vi "plot_example_XY.vi"() -> ()   [LabVIEW 2010, in "OSA.lvclass"]
doc: "Example for plotting XY data, with data reduction, (10E6 XY pairs reduced to graph pixel X-size)."
uses:
  OSA.lvclass
  <vilib>/measure/NI_MABase.lvlib
  typeDef/acq_dataType.ctl
  _misc/Thorlabs_FTS_misc.llb/graph_spectrum.ctl
  OSA20X_misc.lvlib
panel:
  in  "exit butt":bool
  in  "ZOOM OUT BUTTON":bool
  in  "PANE RIGHT":bool
  in  "PANE LEFT":bool
  in  "ZOOM RESTORE":bool
  in  "ZOOM IN BUTTON":bool
  out "Intensity Graph spectrum":T1
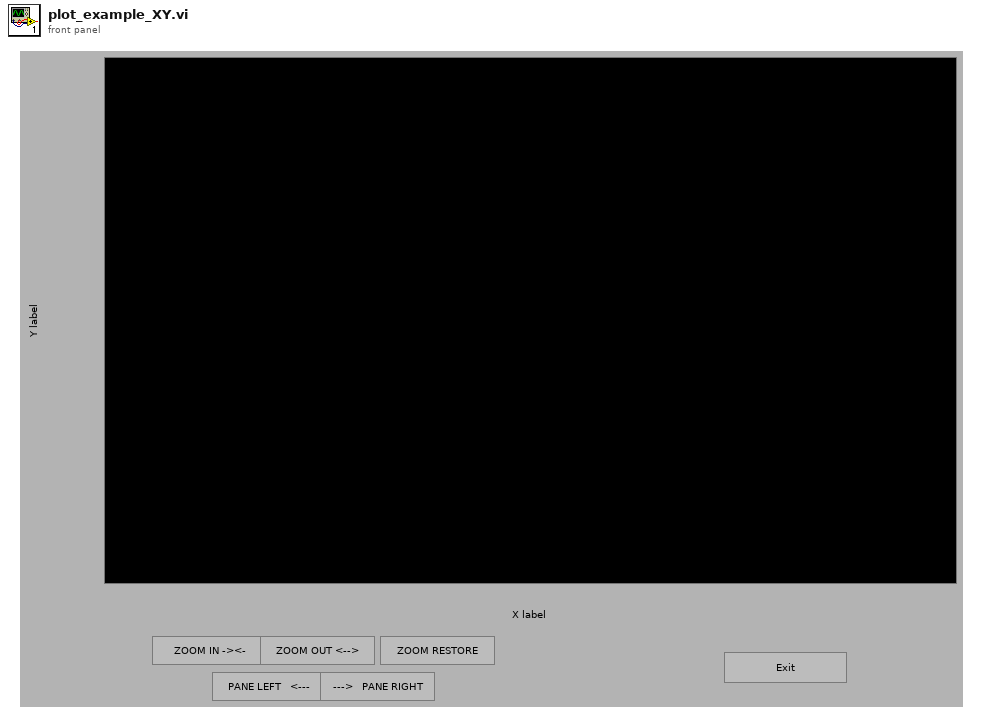
[diagram p1: front panel]
types:
  T1 = typedef "OSA20X_misc.lvlib/graph_spectrum.ctl" = i32[][]
  T2 = typedef "OSA.lvclass/acq_dataType.ctl" = enum16{"none", "interferogram", "spectrum"}
  T3 = enum16{"user", "cursor", "mouse", "pane", "reset"}
  T4 = enum16{"user", "cursor", "mouse", "pane", "reset", "pane right", "zoom out"}
  T5 = enum16{"user", "cursor", "mouse", "pane", "reset", "pane right"}
  T6 = typedef "LVPoint32TypeDef.ctl" = cluster{"Horizontal":i32, "Vertical":i32}
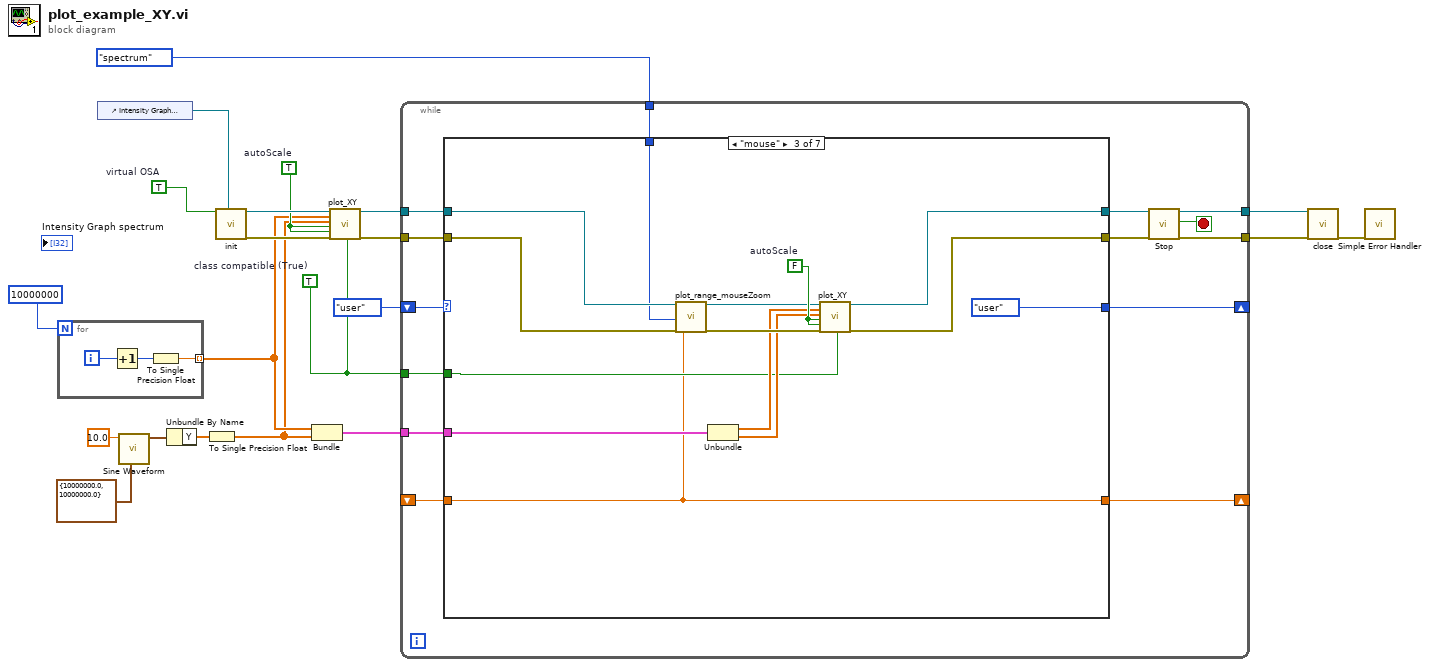
[diagram p0: block diagram]
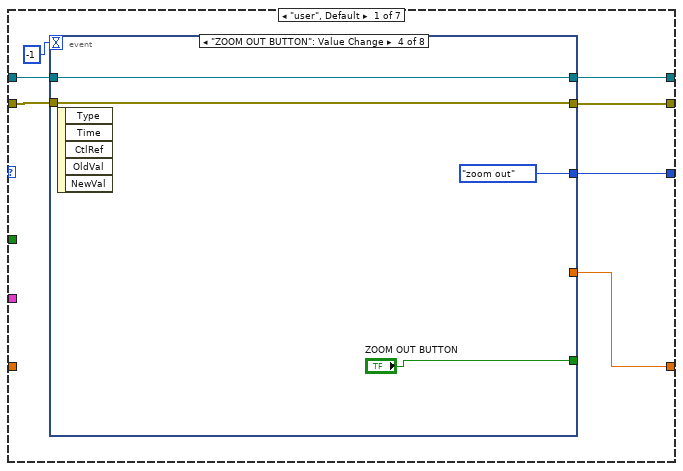
[diagram p2: hidden frame]
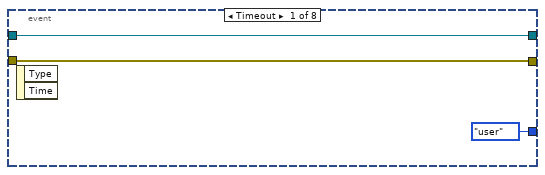
[diagram p3: hidden frame]
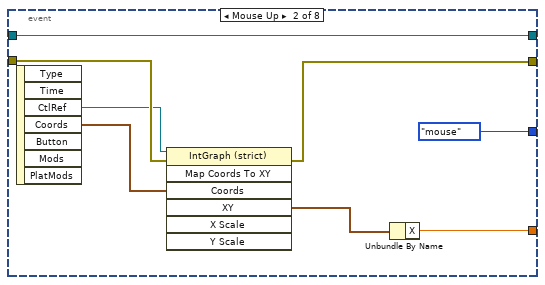
[diagram p4: hidden frame]
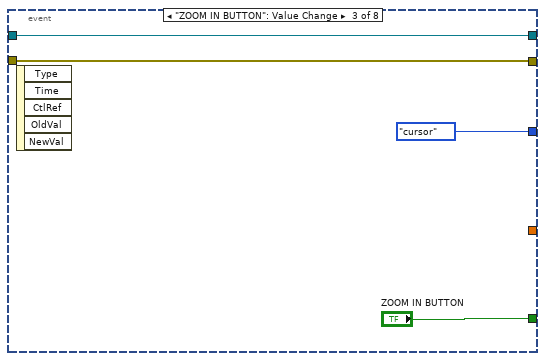
[diagram p5: hidden frame]
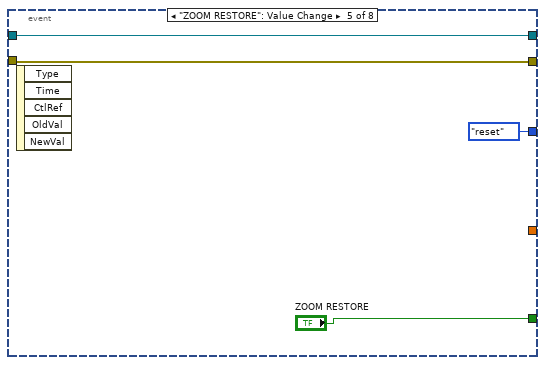
[diagram p6: hidden frame]
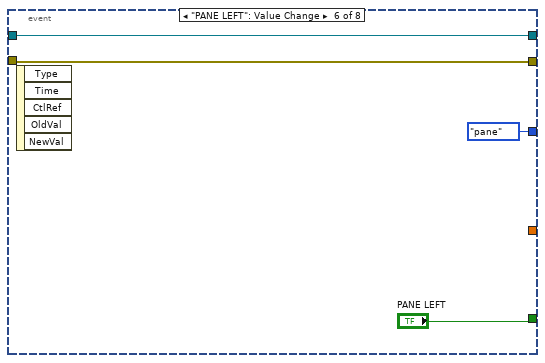
[diagram p7: hidden frame]
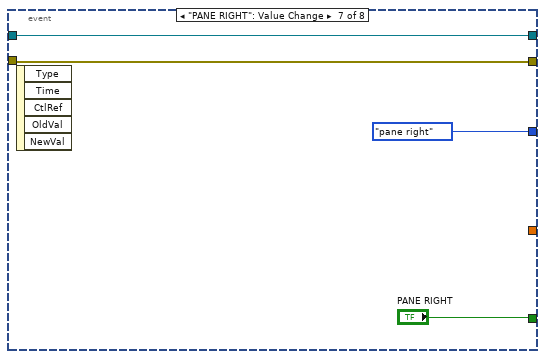
[diagram p8: hidden frame]
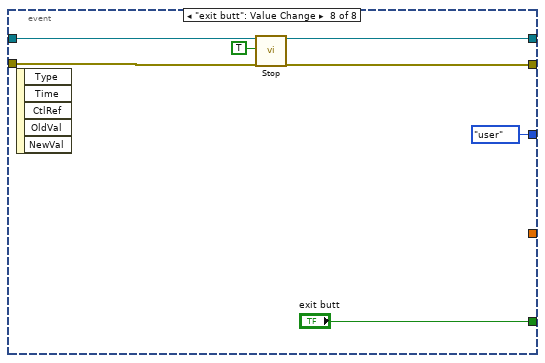
[diagram p9: hidden frame]
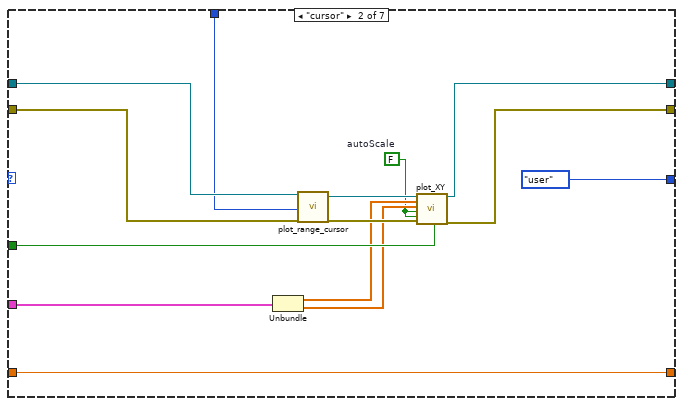
[diagram p10: hidden frame]
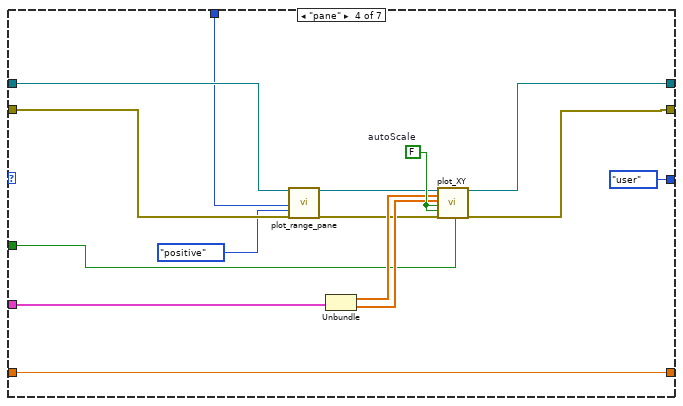
[diagram p11: hidden frame]
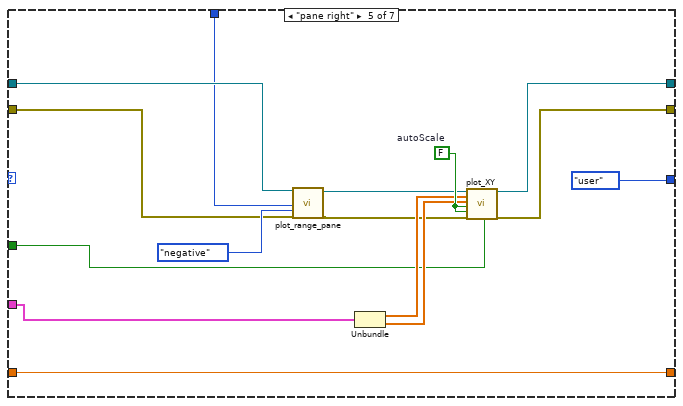
[diagram p12: hidden frame]
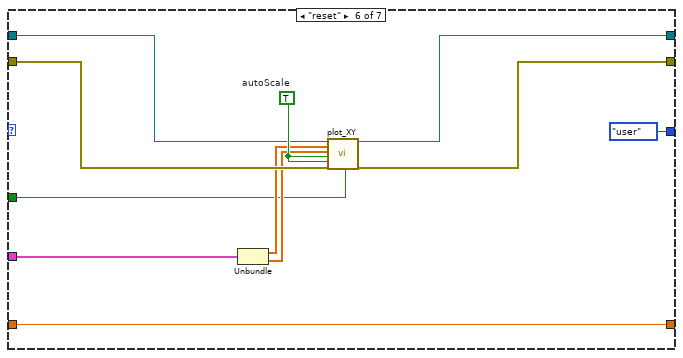
[diagram p13: hidden frame]
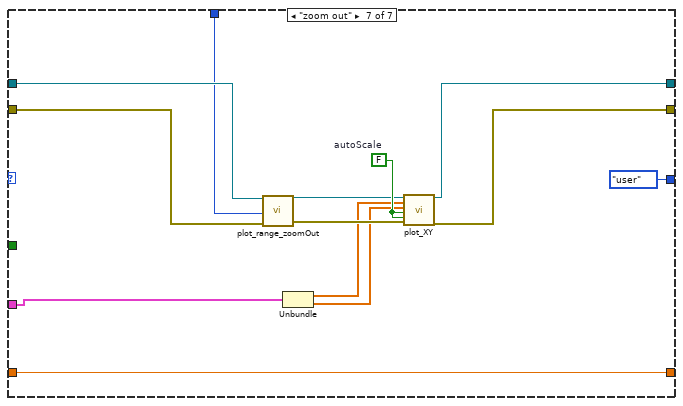
[diagram p14: hidden frame]
diagram:
  w6 = TRUE  # class compatible (True)
  w7 = TRUE  # autoScale
  w19 = TRUE  # virtual OSA
  n1 = for {
    N: 10000000 -> [_]
    tunnel: [w23] -> w5 mode=indexing
    i -> [w24]
    n2 = Increment(x=w24) -> (x+1=w22:i32)
    n3 = To Single Precision Float(number=w22) -> (single precision float=w23:sgl)
  }
  n4 = control-ref of="Intensity Graph spectrum"() -> (w18:refnum<vi>)
  n5 = call <vilib>:"Sine Waveform.vi"("sampling info"=cluster{"Fs":dbl, "#s":dbl} {"Fs"=10000000.0, "#s"=10000000.0}, "frequency"=10.0) -> ("signal out"=w16:waveform(dbl))  [unwired: 8 in, 1 out]
  n6 = Unbundle By Name(w16) -> ("Y"=w12:dbl[])
  n7 = To Single Precision Float(number=w12) -> (single precision float=w4:sgl[])
  n8 = call "init.vi"("virtual OSA"=w19, "Graph Spectrum"=w18) -> ("duplicate reference"=w21:refnum<class "OSA.lvclass">, "error out"=w20:errorcluster)  [unwired: 13 in, 3 out]
  n9 = Bundle(w5, w4) -> (w3:cluster{sgl[], sgl[]})  [unwired: 1 in]
  n10 = call "plot_XY.vi"("reference"=w21, "X-data"=w5, "Y-data"=w4, "autoScale X (True)"=w7, "autoScale Y (True)"=w7, "error in (no error)"=w20, "class compatible (True)"=w6) -> ("duplicate reference"=w11:refnum<class "OSA.lvclass">, "error out"=w10:errorcluster)  [unwired: 11 in]
  n11 = while {
    shift-right: [w37] -> _
    shift-left: T3."user" -> [w38]
    tunnel: w11 -> [w36]
    tunnel: w10 -> [w35]
    tunnel: [w26] -> w9
    tunnel: [w27] -> w8
    tunnel: w6 -> [w34]
    tunnel: w3 -> [w33]
    tunnel: acq_dataType."spectrum" ("dataType") -> [w32]
    shift-right: [w31] -> _
    shift-left: _ -> [w30]
    stop <- w25 stop-if-true
    n12 = case shown="\"mouse\"" w38 {
      tunnel: [w44 T3."user" T3."user" T3."user" T3."user" T5."user" T4."user"] -> w37
      tunnel: w36 -> [w40 w97 w109 w125 w140 w151 w165]
      tunnel: w35 -> [w43 w96 w110 w126 w139 w148 w164]
      tunnel: [w42 w94 w102 w113 w131 w149 w159] -> w28
      tunnel: [w39 w92 w101 w114 w132 w150 w160] -> w29
      tunnel: w34 -> [_ w90 w100 w112 w127 w142 _]
      tunnel: w33 -> [_ w91 w105 w117 w128 w147 w156]
      tunnel: w32 -> [_ w85 w106 w123 w138 _ w162]
      tunnel: [w41 w84 w98 w121 w137 w143 w153] -> w31
      tunnel: w30 -> [_ w84 w98 w121 w137 w143 w153]
      frame "user", Default {
        n13 = event shown="[3] \"ZOOM OUT BUTTON\": Value Change" {
          selector: _ -> [_ _ _ _ _ _ _ _]
          dyn-events: _ -> [_ _ _ _ _ _ _ _]
          timeout: -1 -> [_ _ _ _ _ _ _ _]
          tunnel: [T3."user" T3."mouse" T3."cursor" T4."zoom out" T5."reset" T3."pane" T5."pane right" T3."user"] -> w44
          tunnel: w43 -> [w47 w54 w59 w63 w65 w70 w74 w82]
          tunnel: [w47 w53 w59 w63 w65 w70 w74 w81] -> w42
          tunnel: [_ w51 _ _ _ _ _ _] -> w41
          tunnel: w40 -> [w46 w49 w58 w62 w66 w71 w75 w83]
          tunnel: [w46 w49 w58 w62 w66 w71 w75 w80] -> w39
          tunnel: [_ _ "ZOOM IN BUTTON" "ZOOM OUT BUTTON" "ZOOM RESTORE" "PANE LEFT" "PANE RIGHT" "exit butt"] -> _
          event Timeout {
            n14 = event-data() -> ()  [unwired: 1 in, 2 out]
          }
          event Mouse Up {
            n15 = event-data() -> ("CtlRef"=w50:refnum<vi>, "Coords"=w55:T6)  [unwired: 1 in, 5 out]
            n16 = invoke class="IntGraph (strict)" method="Map Coords To XY"(reference=w50, error in=w54, "Coords"=w55) -> (error out=w53:errorcluster, "XY"=w52:cluster{"X":dbl, "Y":dbl})  [unwired: 4 in, 5 out]
            n17 = Unbundle By Name(w52) -> ("X"=w51:dbl)
          }
          event "ZOOM IN BUTTON": Value Change {
            n18 = event-data() -> ()  [unwired: 1 in, 5 out]
          }
          event "ZOOM OUT BUTTON": Value Change {
            n19 = event-data() -> ()  [unwired: 1 in, 5 out]
          }
          event "ZOOM RESTORE": Value Change {
            n20 = event-data() -> ()  [unwired: 1 in, 5 out]
          }
          event "PANE LEFT": Value Change {
            n21 = event-data() -> ()  [unwired: 1 in, 5 out]
          }
          event "PANE RIGHT": Value Change {
            n22 = event-data() -> ()  [unwired: 1 in, 5 out]
          }
          event "exit butt": Value Change {
            n23 = event-data() -> ()  [unwired: 1 in, 5 out]
            n24 = call "Stop.vi"("reference"=w83, "Stop"=TRUE, "error in (no error)"=w82) -> ("reference"=w80:refnum<class "OSA.lvclass">, "error out"=w81:errorcluster)  [unwired: 14 in, 1 out]
          }
        }
      }
      frame "cursor" {
        w86 = FALSE  # autoScale
        n25 = Unbundle(w91) -> (w89:sgl[], w88:sgl[])
        n26 = call "plot_range_cursor.vi"("reference"=w97, "dataType"=w85, "error in (no error)"=w96) -> ("duplicate reference"=w93:refnum<class "OSA.lvclass">, "error out"=w95:errorcluster)  [unwired: 15 in]
        n27 = call "plot_XY.vi"("reference"=w93, "X-data"=w89, "Y-data"=w88, "autoScale X (True)"=w86, "autoScale Y (True)"=w86, "error in (no error)"=w95, "class compatible (True)"=w90) -> ("duplicate reference"=w92:refnum<class "OSA.lvclass">, "error out"=w94:errorcluster)  [unwired: 11 in]
      }
      frame "mouse" {
        w111 = FALSE  # autoScale
        n28 = call "plot_range_mouseZoom.vi"("reference"=w109, "dataType"=w106, "error in (no error)"=w110, "X mouse"=w98) -> ("duplicate reference"=w107:refnum<class "OSA.lvclass">, "error out"=w108:errorcluster)  [unwired: 14 in]
        n29 = Unbundle(w105) -> (w104:sgl[], w103:sgl[])
        n30 = call "plot_XY.vi"("reference"=w107, "X-data"=w104, "Y-data"=w103, "autoScale X (True)"=w111, "autoScale Y (True)"=w111, "error in (no error)"=w108, "class compatible (True)"=w100) -> ("duplicate reference"=w101:refnum<class "OSA.lvclass">, "error out"=w102:errorcluster)  [unwired: 11 in]
      }
      frame "pane" {
        w120 = FALSE  # autoScale
        n31 = call "plot_range_pane.vi"("reference"=w125, "dataType"=w123, "direction"=enum16{"positive", "negative"}."positive", "error in (no error)"=w126) -> ("duplicate reference"=w115:refnum<class "OSA.lvclass">, "error out"=w116:errorcluster)  [unwired: 14 in]
        n32 = Unbundle(w117) -> (w119:sgl[], w118:sgl[])
        n33 = call "plot_XY.vi"("reference"=w115, "X-data"=w119, "Y-data"=w118, "autoScale X (True)"=w120, "autoScale Y (True)"=w120, "error in (no error)"=w116, "class compatible (True)"=w112) -> ("duplicate reference"=w114:refnum<class "OSA.lvclass">, "error out"=w113:errorcluster)  [unwired: 11 in]
      }
      frame "pane right" {
        w135 = FALSE  # autoScale
        n34 = call "plot_range_pane.vi"("reference"=w140, "dataType"=w138, "direction"=enum16{"positive", "negative"}."negative", "error in (no error)"=w139) -> ("duplicate reference"=w130:refnum<class "OSA.lvclass">, "error out"=w129:errorcluster)  [unwired: 14 in]
        n35 = Unbundle(w128) -> (w134:sgl[], w133:sgl[])
        n36 = call "plot_XY.vi"("reference"=w130, "X-data"=w134, "Y-data"=w133, "autoScale X (True)"=w135, "autoScale Y (True)"=w135, "error in (no error)"=w129, "class compatible (True)"=w127) -> ("duplicate reference"=w132:refnum<class "OSA.lvclass">, "error out"=w131:errorcluster)  [unwired: 11 in]
      }
      frame "reset" {
        w152 = TRUE  # autoScale
        n37 = Unbundle(w147) -> (w146:sgl[], w145:sgl[])
        n38 = call "plot_XY.vi"("reference"=w151, "X-data"=w146, "Y-data"=w145, "autoScale X (True)"=w152, "autoScale Y (True)"=w152, "error in (no error)"=w148, "class compatible (True)"=w142) -> ("duplicate reference"=w150:refnum<class "OSA.lvclass">, "error out"=w149:errorcluster)  [unwired: 11 in]
      }
      frame "zoom out" {
        w161 = FALSE  # autoScale
        n39 = call "plot_range_zoomOut.vi"("reference"=w165, "dataType"=w162, "error in (no error)"=w164) -> ("duplicate reference"=w157:refnum<class "OSA.lvclass">, "error out"=w158:errorcluster)  [unwired: 15 in]
        n40 = Unbundle(w156) -> (w155:sgl[], w154:sgl[])
        n41 = call "plot_XY.vi"("reference"=w157, "X-data"=w155, "Y-data"=w154, "autoScale X (True)"=w161, "autoScale Y (True)"=w161, "error in (no error)"=w158) -> ("duplicate reference"=w160:refnum<class "OSA.lvclass">, "error out"=w159:errorcluster)  [unwired: 12 in]
      }
    }
    n42 = call "Stop.vi"("reference"=w29, "error in (no error)"=w28) -> ("reference"=w27:refnum<class "OSA.lvclass">, "Stop"=w25:bool, "error out"=w26:errorcluster)  [unwired: 15 in]
  }
  n43 = call "close.vi"("reference"=w8, "error in (no error)"=w9) -> ("error out"=w1:errorcluster)  [unwired: 17 in]
  n44 = call <vilib>:"Simple Error Handler.vi"("error in (no error)"=w1) -> ()  [unwired: 4 in, 5 out]
